vi "InitChartFrameIn.vi"(11 "PictureIn":picture) -> (3 "PictureOut":picture)   [LabVIEW 2014]
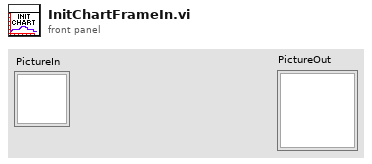
[diagram p1: front panel]
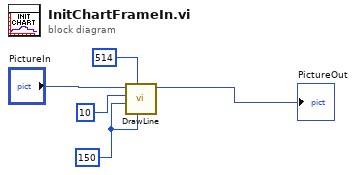
[diagram p0: block diagram]
diagram:
  w2 = i16 150 ("yStart")
  n1 = call "DrawLine.vi"("yEnd"=w2, "xEnd"=i16 514, "yStart"=w2, "xStart"=i16 10, "PictureIn"="PictureIn") -> ("PictureOut"=→"PictureOut":picture)  [unwired: 6 in]
